vi "ARM_GRAVITY_FF.vi"(4 "ArmLength_M":dbl, 6 "Mass_Kg":dbl, 7 "Motor Params":cluster{"Motor Type":T1, "Gear Ratio":dbl}, 9 "FF params":T2={"Kg_Gravity_gain"=0.5, "phi_Equilibrium_phase_Deg"=0.0, "Ks"=0.0}, 10 "ArmSpeed_Dmd_RadPerSec":dbl, 11 "ArmAngle_Dmd_Deg":dbl) -> (2 "FeedForward":dbl)   [LabVIEW 2023]
uses:
  <vilib>/Rock Robotics/WPI/ThirdParty/JAS_Junk/TrajLib/Trajectory_Library.lvlib
  <vilib>/Rock Robotics/WPI/ThirdParty/JAS_Junk/TrajLib/Enum/DCMOTOR_TYPES_ENUM.ctl
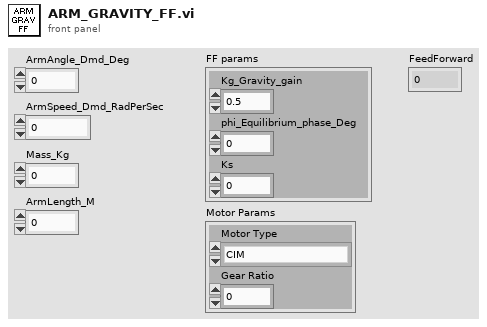
[diagram p1: front panel]
types:
  T1 = typedef "Trajectory_Library.lvlib/DCMOTOR_TYPES_ENUM.ctl" = enum16{"CIM", "AndyMark 9015", "Andy Mark RS 775 125", "Bag", "BaneBots RS 550", "BaneBots RS 775", "Falcon 500", "Mini CIM", "NEO", "NEO 550", "Romi BuiltIn", "Vex 775 Pro", "Snow Blower AM 2235A", "Bosch Seat AM 3493"}
  T2 = cluster{"Kg_Gravity_gain":dbl, "phi_Equilibrium_phase_Deg":dbl, "Ks":dbl}
  T3 = typedef "Trajectory_Library.lvlib/DCMOTOR.CTL" = cluster{"nominalVoltage_Volts":dbl, "StallTorque_NM":dbl, "StallCurrent_Amps":dbl, "FreeCurrent_Amps":dbl, "FreeSpeed_RadPerSec":dbl, "R_Ohms":dbl, "KvINV_RadPerSecPerVolt":dbl, "Kt_NMPerAmp":dbl, "L_H":dbl, "Jr_KgM2":dbl}
  T4 = typedef "Trajectory_Library.lvlib/SIMPLE_MOTOR_FF.ctl" = cluster{"Ks":dbl, "Kv":dbl, "Ka":dbl, "KnInv":dbl}
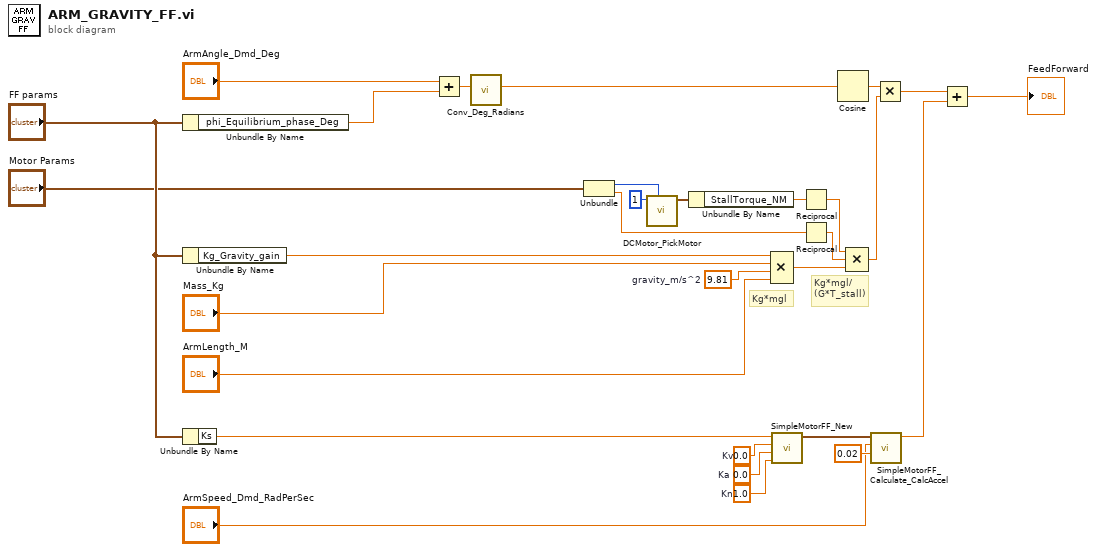
[diagram p0: block diagram]
diagram:
  w23 = 1.0  # Kn
  w22 = 0.0  # Ka
  w21 = 0.0  # Kv
  w12 = 9.81  # gravity_m/s^2
  # "Kg*mgl/\n(G*T_stall)"
  # "Kg*mgl"
  n1 = Unbundle By Name("FF params") -> ("phi_Equilibrium_phase_Deg"=w6:dbl)
  n2 = Unbundle By Name("FF params") -> ("Kg_Gravity_gain"=w4:dbl)
  n3 = Unbundle By Name("FF params") -> ("Ks"=w5:dbl)
  n4 = Add(x="ArmAngle_Dmd_Deg", y=w6) -> (x+y=w14:dbl)
  n5 = call <vilib>:"Conv_Deg_Radians.vi"("Degress"=w14) -> ("Radians"=w15:dbl)  [unwired: 10 in]
  n6 = Unbundle("Motor Params") -> ("Motor Type"=w26:T1, "Gear Ratio"=w27:dbl)
  n7 = call <vilib>:"DCMotor_PickMotor.vi"("DCMOTOR_TYPES"=w26, "Num Motors"=1) -> ("DCMOTOR"=w10:T3)  [unwired: 9 in]
  n8 = Unbundle By Name(w10) -> ("StallTorque_NM"=w28:dbl)
  n9 = Compound Arithmetic op=MULTIPLY(w4, "Mass_Kg", w12, "ArmLength_M") -> (w11:dbl)
  n10 = call <vilib>:"SimpleMotorFF_New.vi"("Kn"=w23, "Ka"=w22, "Kv"=w21, "Ks"=w5) -> ("SIMPLE_MOTOR_FF"=w24:T4)  [unwired: 7 in]
  n11 = Reciprocal(x=w28) -> (1/x=w25:dbl)
  n12 = Reciprocal(x=w27) -> (1/x=w13:dbl)
  n13 = Cosine(x=w15) -> (cos(x)=w8:dbl)
  n14 = Compound Arithmetic op=MULTIPLY(w25, w13, w11) -> (w7:dbl)
  n15 = call <vilib>:"SimpleMotorFF_Calculate_CalcAccel.vi"("dT_Sec"=0.02, "VelSp"="ArmSpeed_Dmd_RadPerSec", "SIMPLE_MOTOR_FF"=w24) -> ("FeedForward"=w19:dbl)  [unwired: 8 in]
  n16 = Multiply(x=w8, y=w7) -> (x*y=w18:dbl)
  n17 = Add(x=w18, y=w19) -> (x+y=→"FeedForward":dbl)
